vi "Lab18_motorControl.vi"() -> ()   [LabVIEW 2022 SP3]
uses:
  Lab18_servoStates.ctl
  <vilib>/DAQmx/create/channels.llb/DAQmx Create Channel (CO-Pulse Generation-Time).vi
  <vilib>/DAQmx/configure/timing.llb/DAQmx Timing (Implicit).vi
  <resource>/objmgr/daqmx.rc
panel:
  out "Current State":T1
  in  "Right Speed":dbl=1.3 step=1e-05 format="%#_6p"
  in  "Left Speed":dbl=1.7 step=1e-05 format="%#_6p"
  in  "Motor Direction":bool
  in  "CO.Pulse.Term":tag="/Dev1/PFI0"
  in  "Motor Speed":u16(ring)=3 items=["Fast", "Medium", "Slow", "Rest"]
  out "Pulse Time":dbl=0.0015 format="%#_6p"
  in  "stop":bool
  in  "Tab Control":enum32{"Finite", "Continuous"}(tab)=enum."Continuous"
  in  "# of Pulses":i32=100 min=1
  in  "Finite Start":bool
  in  "Continuous Start":bool
  in  "counter":tag="Dev1/ctr0"
  # "Left"
  # "Right"
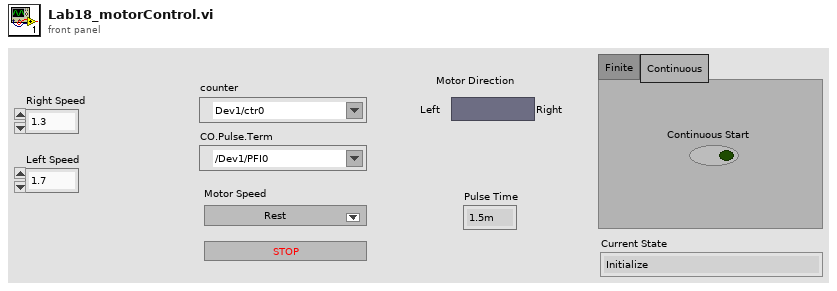
[diagram p1: front panel]
types:
  T1 = typedef "Lab18_servoStates.ctl" = enum16{"Initialize", "ModeSelect", "MainState", "Stop", "Finite", "Continuous", "UpdateSpeed"}
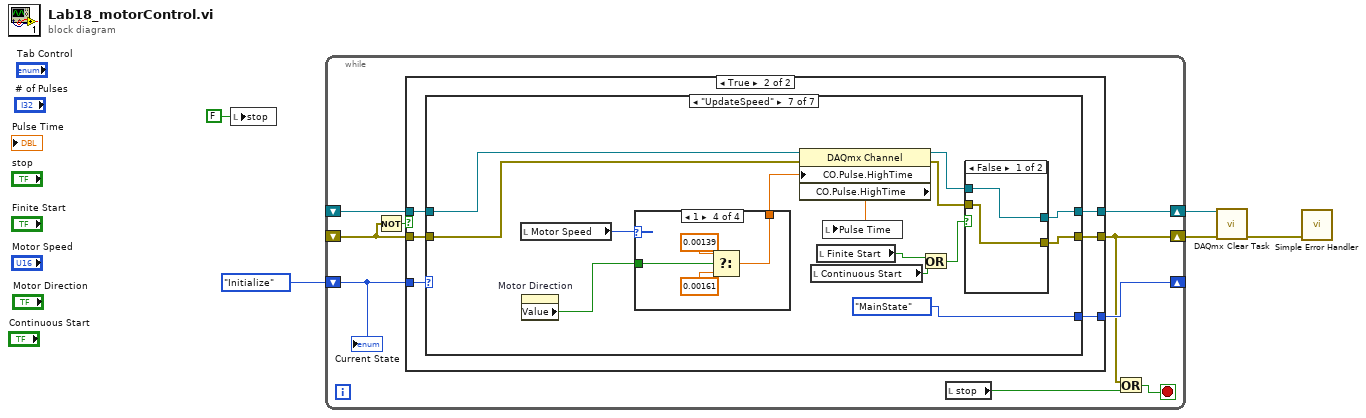
[diagram p0: block diagram]
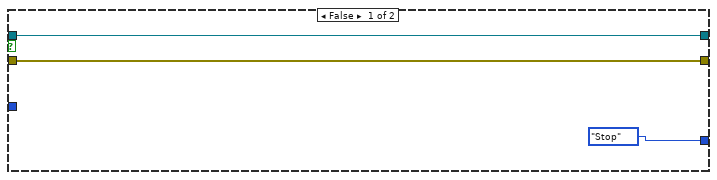
[diagram p2: hidden frame]
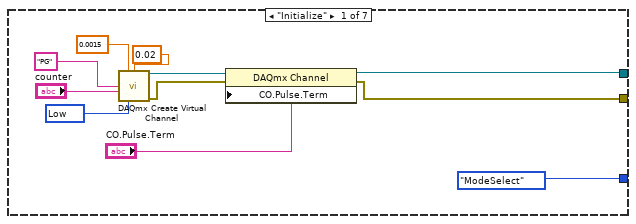
[diagram p3: hidden frame]
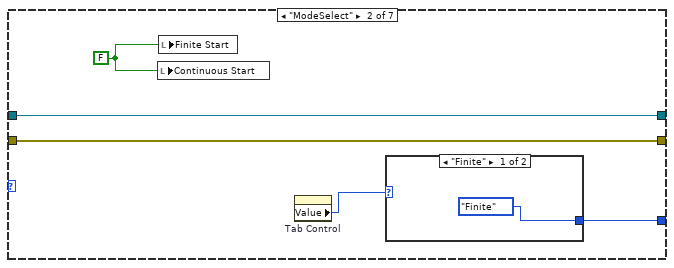
[diagram p4: hidden frame]
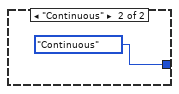
[diagram p5: hidden frame]
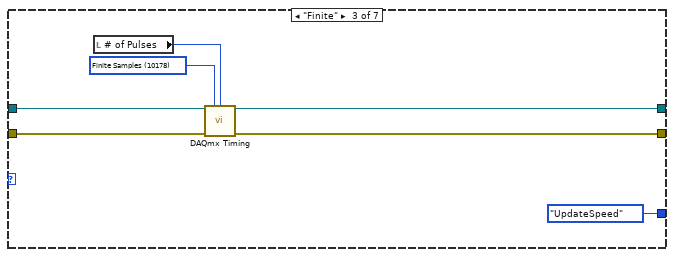
[diagram p6: hidden frame]
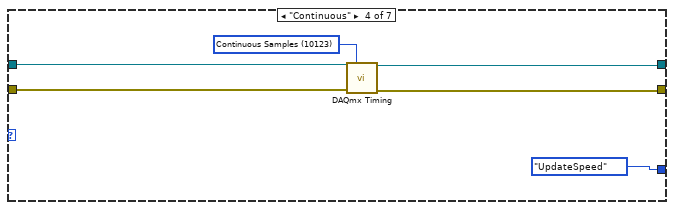
[diagram p7: hidden frame]
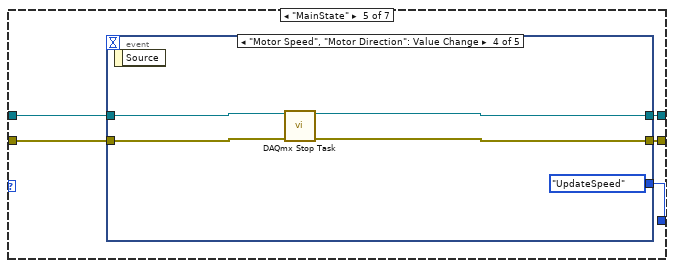
[diagram p8: hidden frame]
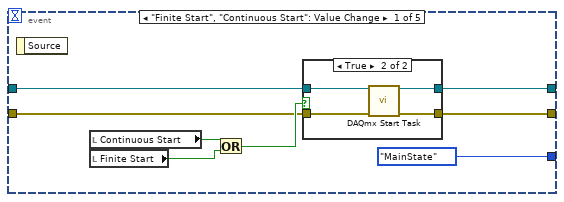
[diagram p9: hidden frame]
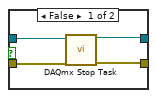
[diagram p10: hidden frame]
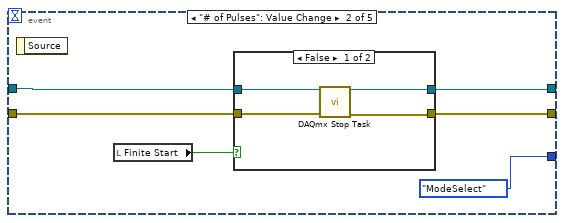
[diagram p11: hidden frame]
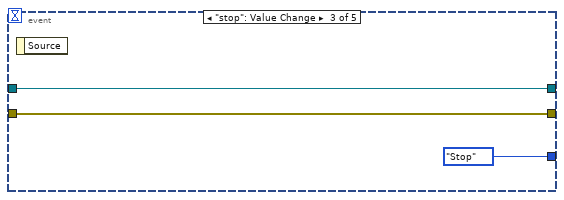
[diagram p13: hidden frame]
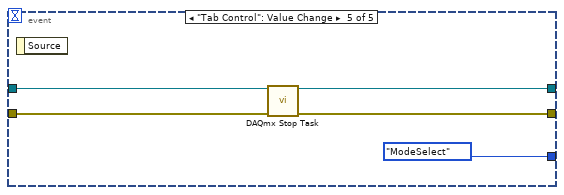
[diagram p14: hidden frame]
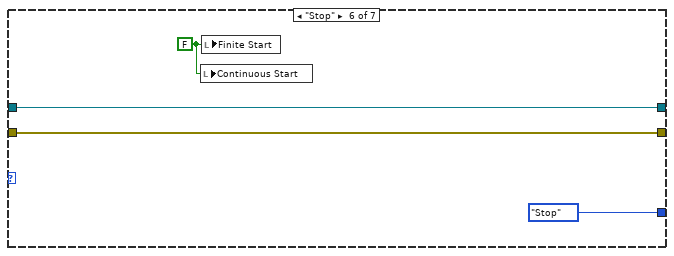
[diagram p15: hidden frame]
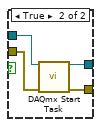
[diagram p16: hidden frame]
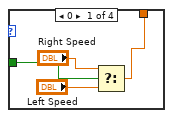
[diagram p17: hidden frame]
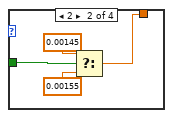
[diagram p18: hidden frame]
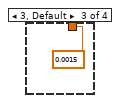
[diagram p19: hidden frame]
diagram:
  n1 = local write "stop"(FALSE ("stop")) -> ()
  n2 = while {
    shift-right: [w13] -> _
    shift-left: Lab18_servoStates."Initialize" -> [w12]
    shift-right: [w14] -> w3
    shift-left: _ -> [w11]
    shift-right: [w7] -> w2
    shift-left: _ -> [w9]
    stop <- w8 stop-if-true
    n3 = Not(x=w9) -> (.not. x?=w10:bool)
    n4 = case shown="True" w10 {
      tunnel: [w17 w23] -> w14
      tunnel: [w16 w22] -> w7
      tunnel: [Lab18_servoStates."Stop" w21] -> w13
      tunnel: w12 -> [_ w20]
      tunnel: w11 -> [w17 w19]
      tunnel: w9 -> [w16 w18]
      frame False {
      }
      frame True {
        n5 = case shown="\"UpdateSpeed\"" w20 {
          tunnel: [w28 w38 w45 w50 w56 w103 w107] -> w23
          tunnel: [w27 w37 w44 w51 w55 w102 w105] -> w22
          tunnel: [Lab18_servoStates."ModeSelect" w35 Lab18_servoStates."UpdateSpeed" Lab18_servoStates."UpdateSpeed" w57 Lab18_servoStates."Stop" Lab18_servoStates."MainState"] -> w21
          tunnel: w19 -> [_ w38 w47 w53 w59 w103 w114]
          tunnel: w18 -> [_ w37 w46 w52 w58 w102 w113]
          frame "Initialize" {
            w31 = 10214 items=["High"=10192, "Low"=10214] ("idle state")
            n6 = call-poly <vilib>:"DAQmx Create Virtual Channel.vi"("high time"=0.0015, "low time"=0.02, "counter"="counter", "name to assign"="PG", "idle state"=w31) -> ("task out"=w30:refnum<k21>, "error out"=w29:errorcluster)  [unwired: 9 in]
            n7 = property class="DAQmx Channel"(reference=w30, error in=w29, "CO.Pulse.Term"="CO.Pulse.Term") -> (reference out=w28:refnum<k21>, error out=w27:errorcluster)
          }
          frame "ModeSelect" {
            w39 = FALSE ("Finite Start")
            n8 = local write "Continuous Start"(w39) -> ()
            n9 = local write "Finite Start"(w39) -> ()
            n10 = property on="Tab Control" class="TabCtl (strict)"() -> ("Value"=w36:enum32{"Finite", "Continuous"})  [unwired: 2 in, 2 out]
            n11 = case shown="\"Finite\"" w36 {
              tunnel: [Lab18_servoStates."Finite" Lab18_servoStates."Continuous"] -> w35
              frame "Finite" {
              }
              frame "Continuous" {
              }
            }
          }
          frame "Finite" {
            w48 = 10178 items=["Finite Samples"=10178, "Continuous Samples"=10123, "Hardware Timed Single Point"=12522] ("sample mode")
            n12 = local read "# of Pulses"() -> (w42:i32)
            n13 = call-poly <vilib>:"DAQmx Timing.vi"("task/channels in"=w47, "sample mode"=w48, "samples per channel"=w42, "error in"=w46) -> ("task out"=w45:refnum<k21>, "error out"=w44:errorcluster)  [unwired: 10 in]
          }
          frame "Continuous" {
            w54 = 10123 items=["Finite Samples"=10178, "Continuous Samples"=10123, "Hardware Timed Single Point"=12522] ("sample mode")
            n14 = call-poly <vilib>:"DAQmx Timing.vi"("task/channels in"=w53, "sample mode"=w54, "error in"=w52) -> ("task out"=w50:refnum<k21>, "error out"=w51:errorcluster)  [unwired: 11 in]
          }
          frame "MainState" {
            n15 = event shown="[3] \"Motor Speed\", \"Motor Direction\": Value Change" {
              selector: _ -> [_ _ _ _ _]
              dyn-events: _ -> [_ _ _ _ _]
              timeout: _ -> [_ _ _ _ _]
              tunnel: w59 -> [w63 w80 w90 w94 w99]
              tunnel: w58 -> [w62 w79 w89 w93 w98]
              tunnel: [Lab18_servoStates."MainState" Lab18_servoStates."ModeSelect" Lab18_servoStates."Stop" Lab18_servoStates."UpdateSpeed" Lab18_servoStates."ModeSelect"] -> w57
              tunnel: [w61 w77 w90 w92 w96] -> w56
              tunnel: [w60 w78 w89 w91 w97] -> w55
              event "Finite Start", "Continuous Start": Value Change {
                n16 = event-data() -> ()  [unwired: 1 in, 1 out]
                n17 = local read "Continuous Start"() -> (w66:bool)
                n18 = local read "Finite Start"() -> (w65:bool)
                n19 = Or(x=w66, y=w65) -> (x .or. y?=w64:bool)
                n20 = case shown="True" w64 {
                  tunnel: w63 -> [w71 w75]
                  tunnel: w62 -> [w70 w74]
                  tunnel: [w68 w73] -> w61
                  tunnel: [w69 w72] -> w60
                  frame False {
                    n21 = call <vilib>:"DAQmx Stop Task.vi"("task/channels in"=w71, "error in"=w70) -> ("task out"=w68:refnum<k21>, "error out"=w69:errorcluster)  [unwired: 12 in]
                  }
                  frame True {
                    n22 = call <vilib>:"DAQmx Start Task.vi"("task/channels in"=w75, "error in"=w74) -> ("task out"=w73:refnum<k21>, "error out"=w72:errorcluster)  [unwired: 12 in]
                  }
                }
              }
              event "# of Pulses": Value Change {
                n23 = event-data() -> ()  [unwired: 1 in, 1 out]
                n24 = local read "Finite Start"() -> (w81:bool)
                n25 = case shown="False" w81 {
                  tunnel: [w82 w87] -> w77
                  tunnel: w80 -> [w85 w87]
                  tunnel: [w83 w86] -> w78
                  tunnel: w79 -> [w84 w86]
                  frame False {
                    n26 = call <vilib>:"DAQmx Stop Task.vi"("task/channels in"=w85, "error in"=w84) -> ("task out"=w82:refnum<k21>, "error out"=w83:errorcluster)  [unwired: 12 in]
                  }
                  frame True {
                  }
                }
              }
              event "stop": Value Change {
                n27 = event-data() -> ()  [unwired: 1 in, 1 out]
              }
              event "Motor Speed", "Motor Direction": Value Change {
                n28 = event-data() -> ()  [unwired: 1 in, 1 out]
                n29 = call <vilib>:"DAQmx Stop Task.vi"("task/channels in"=w94, "error in"=w93) -> ("task out"=w92:refnum<k21>, "error out"=w91:errorcluster)  [unwired: 12 in]
              }
              event "Tab Control": Value Change {
                n30 = event-data() -> ()  [unwired: 1 in, 1 out]
                n31 = call <vilib>:"DAQmx Stop Task.vi"("task/channels in"=w99, "error in"=w98) -> ("task out"=w96:refnum<k21>, "error out"=w97:errorcluster)  [unwired: 12 in]
              }
            }
          }
          frame "Stop" {
            w101 = FALSE ("Finite Start")
            n32 = local write "Continuous Start"(w101) -> ()
            n33 = local write "Finite Start"(w101) -> ()
          }
          frame "UpdateSpeed" {
            n34 = local read "Motor Speed"() -> (w117:u16)
            n35 = property on="Motor Direction" class="Bool (strict)"() -> ("Value"=w118:bool)  [unwired: 2 in, 2 out]
            n36 = case shown="1" w117 {
              tunnel: [w125 w129 0.0015 w134] -> w116
              tunnel: w118 -> [w126 w131 _ w135]
              frame 0 {
                n37 = Select(t="Right Speed", s=w126, f="Left Speed") -> (s? t:f=w125:dbl)
              }
              frame 2 {
                n38 = Select(t=0.00145, s=w131, f=0.00155) -> (s? t:f=w129:dbl)
              }
              frame 3, Default {
              }
              frame 1 {
                n39 = Select(t=0.00139, s=w135, f=0.00161) -> (s? t:f=w134:dbl)
              }
            }
            n40 = property class="DAQmx Channel"(reference=w114, error in=w113, "CO.Pulse.HighTime"=w116) -> (reference out=w108:refnum<k21>, error out=w106:errorcluster, "CO.Pulse.HighTime"=w115:dbl)
            n41 = local read "Continuous Start"() -> (w110:bool)
            n42 = local read "Finite Start"() -> (w111:bool)
            n43 = local write "Pulse Time"(w115) -> ()
            n44 = Or(x=w111, y=w110) -> (x .or. y?=w109:bool)
            n45 = case shown="False" w109 {
              tunnel: w108 -> [w120 w124]
              tunnel: [w120 w123] -> w107
              tunnel: w106 -> [w119 w122]
              tunnel: [w119 w121] -> w105
              frame False {
              }
              frame True {
                n46 = call <vilib>:"DAQmx Start Task.vi"("task/channels in"=w124, "error in"=w122) -> ("task out"=w123:refnum<k21>, "error out"=w121:errorcluster)  [unwired: 12 in]
              }
            }
          }
        }
      }
    }
    n47 = local read "stop"() -> (w6:bool)
    n48 = Or(x=w7, y=w6) -> (x .or. y?=w8:bool)
    "Current State" <- w12
  }
  n49 = call <vilib>:"DAQmx Clear Task.vi"("task in"=w3, "error in"=w2) -> ("error out"=w4:errorcluster)  [unwired: 13 in]
  n50 = call <vilib>:"Simple Error Handler.vi"("error in (no error)"=w4) -> ()  [unwired: 4 in, 5 out]
